vi "Pre Launch Init.vi"(11 "ModelGeneratesError in":refnum<class "ModelLaunchesActor.lvclass">) -> (0 "error out":errorcluster, 3 "ModelGeneratesError out":refnum<class "ModelLaunchesActor.lvclass">)   [LabVIEW 2017, in "ModelLaunchesActor.lvclass"]
doc: "(<B>Filename</B>: Actor Framework.lvlib:Actor.lvclass:Pre Launch Init.vi)\n\nDefines behavior that occurs after the Launch Nested Actor method is invoked but before the actor's Actor Core method begins running.\n\nBy default, this method does nothing. A descendant class may override it to define behavior."
uses:
  ModelLaunchesActor.lvclass
  C:/Program Files (x86)/National Instruments/LabVIEW 2017/vi.lib/ActorFramework/Actor/Actor.lvclass
  <vilib>/ActorFramework/Message Enqueuer/Message Priority.ctl
  <vilib>/ActorFramework/Actor/Actor.lvclass/Actor.ctl
  <vilib>/ActorFramework/Message Enqueuer/Message Enqueuer.lvclass/Message Enqueuer.ctl
  ModelLaunchesActor.lvclass/ModelLaunchesActor.ctl
  <vilib>/ActorFramework/Message Enqueuer/Init from Existing Queue.vi
  Source/IModel/IModel/IModel.lvclass
  <vilib>/ActorFramework/Message Enqueuer/Message Enqueuer.lvclass
  <vilib>/ActorFramework/Actor/Actor.lvclass
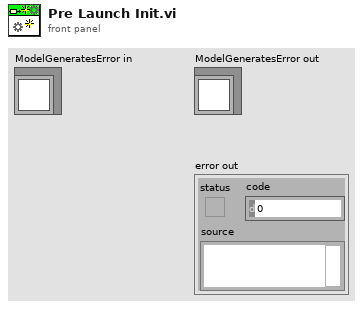
[diagram p1: front panel]
types:
  T1 = typedef "Actor Framework.lvlib/Message Enqueuer.lvclass/Message Priority.ctl" = enum16{"Low", "Normal", "High"}
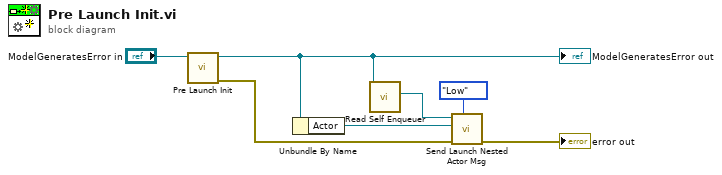
[diagram p0: block diagram]
diagram:
  n1 = call-parent "Pre Launch Init.vi"("IModel in"="ModelGeneratesError in") -> ("error out"=w7:errorcluster, "IModel out"=w1:refnum<class "ModelLaunchesActor.lvclass">)  [unwired: 9 in]
  "ModelGeneratesError out" <- w1
  n2 = Unbundle By Name(w1) -> ("Actor"=w2:refnum<class "Actor.lvclass">)
  n3 = call <vilib>:"Read Self Enqueuer.vi"("Actor"=w1) -> ("Self Enqueuer"=w6:refnum<class "Message Enqueuer.lvclass">)  [unwired: 10 in]
  n4 = call <vilib>:"Send Launch Nested Actor Msg.vi"("Message Priority (Normal)"=Message_Priority."Low", "error in"=w7, "Nested Actor"=w2, "Self Enqueuer in"=w6) -> ("error out"=→"error out":errorcluster)  [unwired: 6 in, 1 out]
